vi "Teleop - Climb System (SubVI).vi"(0 "Driver Climb Activate":bool, 1 "Disabled":bool, 5 "Operator Climb Activate":bool, 7 "Desired cluster In":T3 {"shooterMotorMode" items=["PercentOutput"=0, "Position"=1, "Velocity"=2, "Current"=3, "Follower"=5, "MotionProfile"=6, "MotionMagic"=7, "MotionProfileArc"=10, "Disabled"=15]}, 9 "Constant Cluster in":T2 {"32. shooterHoodAngleRange" format="%_6f"; "31. turretAngleRange" format="%_6f"; "30. shooterVelocityLowerLimit" format="%_6f"; "29. shooterVelocityUpperLimit" format="%_6f"; "28. Robot Track Width (inches)" format="%_6f"; "27. Shooter Spin Up Speed (RPM)" format="%_6f"; "26. Climb Down Speed %" format="%_6f"; "25. Climb Up Speed %" format="%_6f"; "24. wallShooterVelocity" format="%_6f"; "23. Intake Spit Speed %" format="%_6f"; "22. Intake Suck Speed %" format="%_6f"; "21. CP Wheel Diameter" format="%_6f"; "20. Clockwise CP Fudge" format="%_6f"; "19. CouterClockwise CP Fudge" format="%_6f"; "18. Inches per Sector" format="%_6f"; "17. Ticks/Rotation Neo 550" format="%_6f"; "16. Control Panel Wheel Diameter" format="%_6f"; "15. Center-Center Sector Distance" format="%_6f"; "14. Inches / Tick Drivetrain" format="%_6f"; "13. Auton I Output Limit Drive Straight Gain" format="%_6f"; "12. Auton Deriv Drive Straight Gain" format="%_6f"; "11. Auton Int Drive Straight Gain" format="%_6f"; "10. Auton Prop Drive Straight Gain" format="%_6f"; "9. Auton I Output Limit Turn Gain" format="%_6f"; "8. Auton Deriv Turn Gain" format="%_6f"; "7. Auton Int Turn Gain" format="%_6f"; "1. Auton Prop Drive Gain" format="%_6f"; "2. Auton Int Drive Gain" format="%_6f"; "3. Auton Deriv Drive Gain" format="%_6f"; "4. I Output Drive  Limit" format="%_6f"; "5. Auto Drive Cheat (%)" format="%_6f"; "6. Auton Prop Turn Gain" format="%_6f"}, 11 "Climb Up":bool, 12 "Sensors In":T1) -> (8 "Desired cluster Out":T3 {"shooterMotorMode" items=["PercentOutput"=0, "Position"=1, "Velocity"=2, "Current"=3, "Follower"=5, "MotionProfile"=6, "MotionMagic"=7, "MotionProfileArc"=10, "Disabled"=15]}, 10 "Constant Cluster out":T2 {"32. shooterHoodAngleRange" format="%_6f"; "31. turretAngleRange" format="%_6f"; "30. shooterVelocityLowerLimit" format="%_6f"; "29. shooterVelocityUpperLimit" format="%_6f"; "28. Robot Track Width (inches)" format="%_6f"; "27. Shooter Spin Up Speed (RPM)" format="%_6f"; "26. Climb Down Speed %" format="%_6f"; "25. Climb Up Speed %" format="%_6f"; "24. wallShooterVelocity" format="%_6f"; "23. Intake Spit Speed %" format="%_6f"; "22. Intake Suck Speed %" format="%_6f"; "21. CP Wheel Diameter" format="%_6f"; "20. Clockwise CP Fudge" format="%_6f"; "19. CouterClockwise CP Fudge" format="%_6f"; "18. Inches per Sector" format="%_6f"; "17. Ticks/Rotation Neo 550" format="%_6f"; "16. Control Panel Wheel Diameter" format="%_6f"; "15. Center-Center Sector Distance" format="%_6f"; "14. Inches / Tick Drivetrain" format="%_6f"; "13. Auton I Output Limit Drive Straight Gain" format="%_6f"; "12. Auton Deriv Drive Straight Gain" format="%_6f"; "11. Auton Int Drive Straight Gain" format="%_6f"; "10. Auton Prop Drive Straight Gain" format="%_6f"; "9. Auton I Output Limit Turn Gain" format="%_6f"; "8. Auton Deriv Turn Gain" format="%_6f"; "7. Auton Int Turn Gain" format="%_6f"; "1. Auton Prop Drive Gain" format="%_6f"; "2. Auton Int Drive Gain" format="%_6f"; "3. Auton Deriv Drive Gain" format="%_6f"; "4. I Output Drive  Limit" format="%_6f"; "5. Auto Drive Cheat (%)" format="%_6f"; "6. Auton Prop Turn Gain" format="%_6f"}, 14 "Climb is latched":bool, 15 "Sensors Out":T1)   [LabVIEW 2019]
uses:
  Disabled/Constant VI_s/Disabled - Constant Cluster Typedef.ctl
  Autonomous/TypeDefs/Sensor TypeDef.ctl
  Desired Cluster.ctl
  <vilib>/Rock Robotics/WPI/ThirdParty/Phoenix-LabVIEW/Motor Controller/Controls/CTRE_Phoenix_MotorControl_ControlMode.ctl
panel:
  # "Inputs"
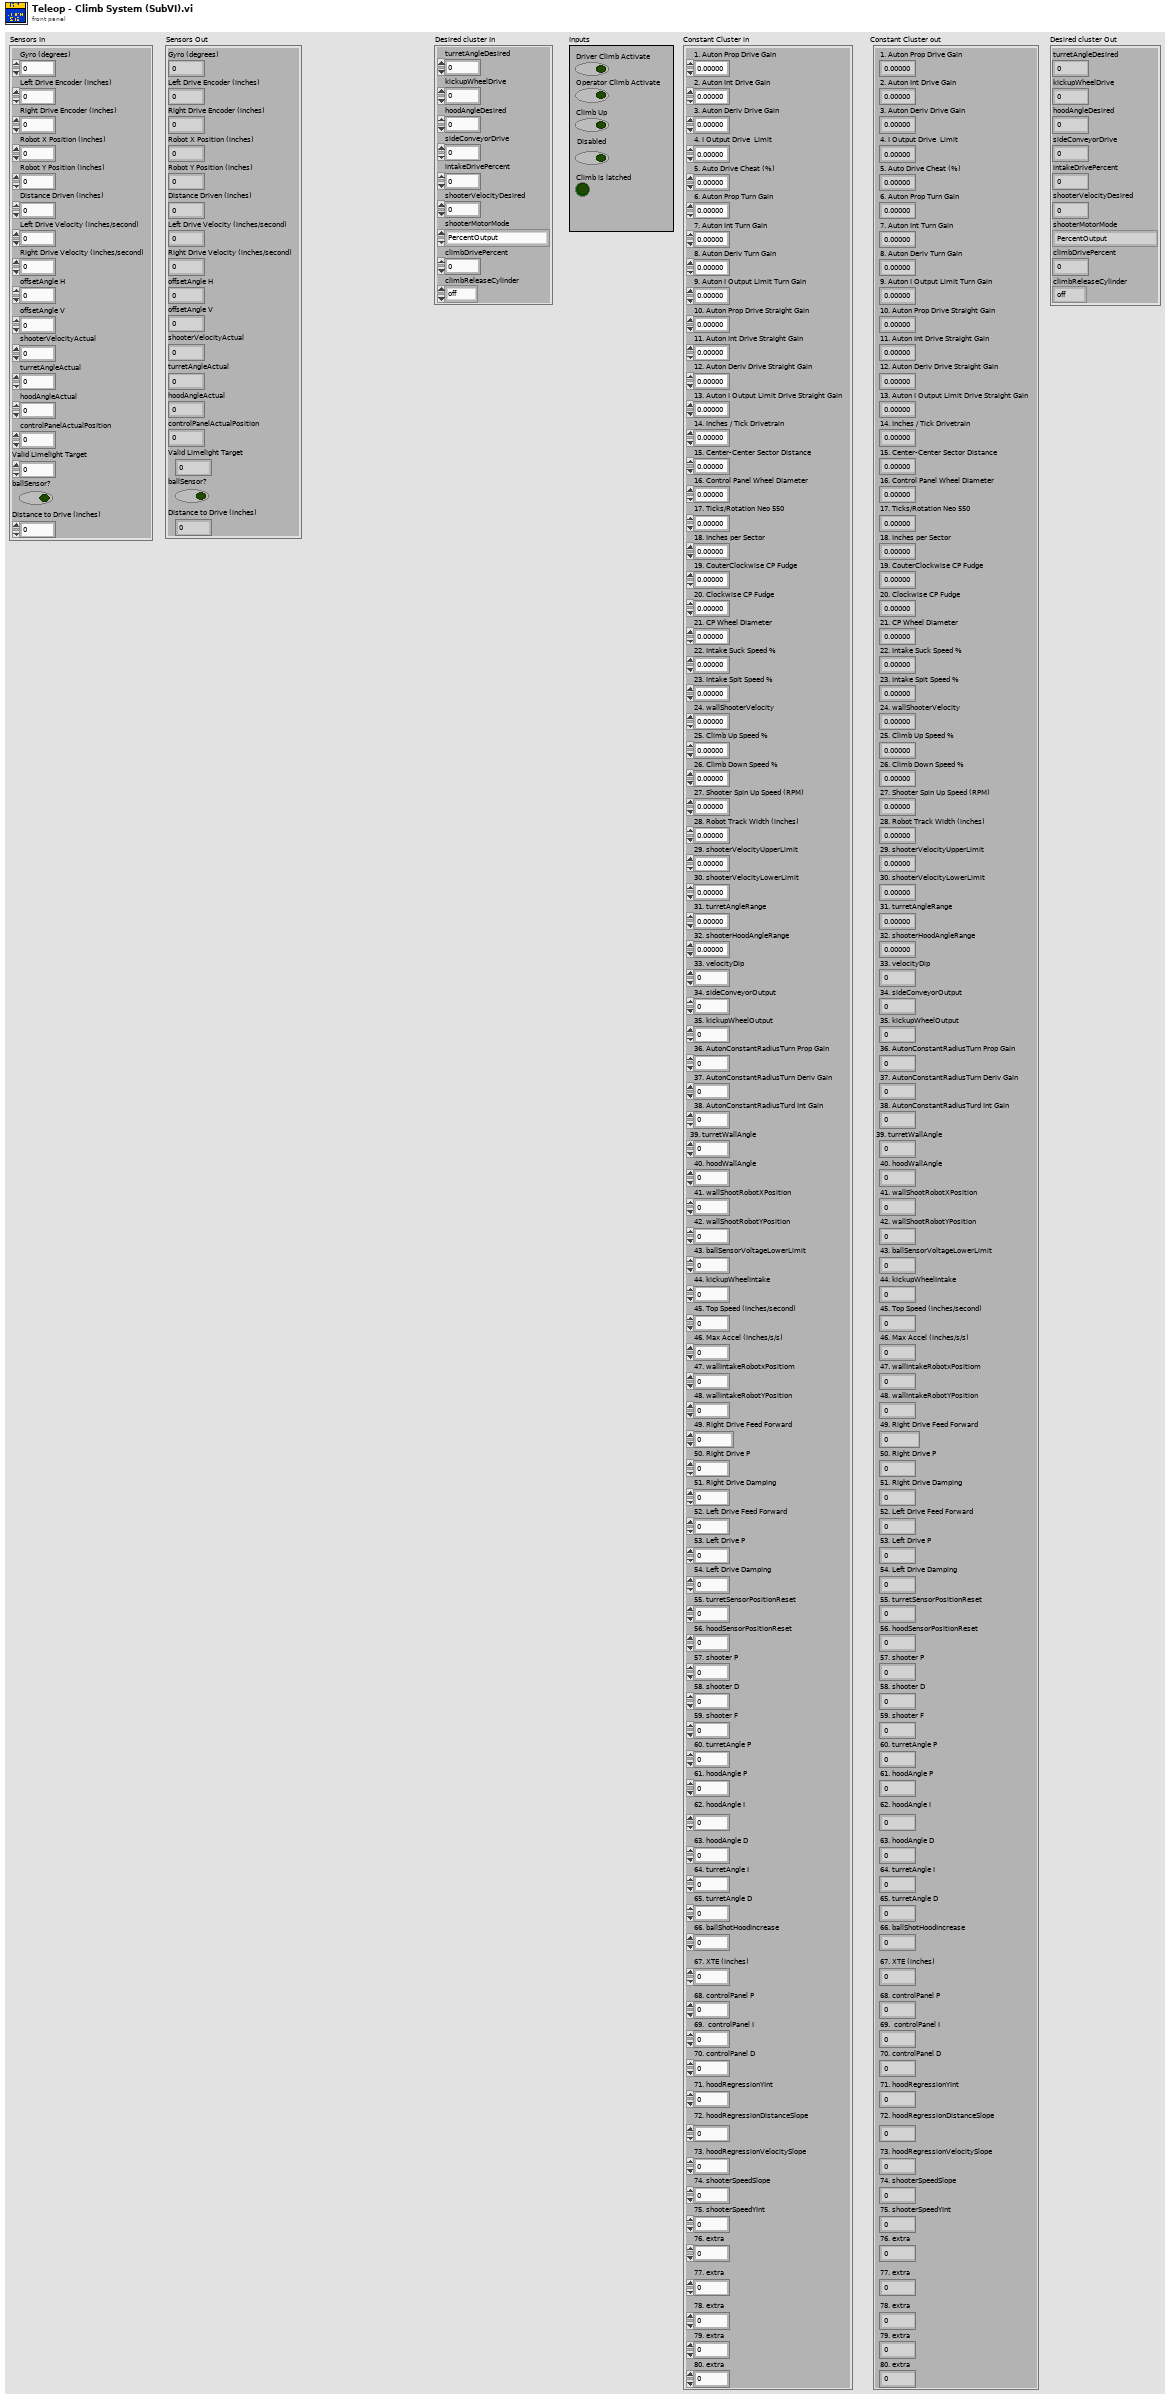
[diagram p1: front panel]
types:
  T1 = typedef "Sensor TypeDef.ctl" = cluster{"Gyro (degrees)":dbl, "Left Drive Encoder (inches)":dbl, "Right Drive Encoder (inches)":dbl, "Robot X Position (inches)":dbl, "Robot Y Position (inches)":dbl, "Distance Driven (inches)":dbl, "Left Drive Velocity (inches/second)":dbl, "Right Drive Velocity (inches/second)":dbl, "offsetAngle H":dbl, "offsetAngle V":dbl, "shooterVelocityActual":dbl, "turretAngleActual":dbl, "hoodAngleActual":dbl, "controlPanelActualPosition":dbl, "Valid Limelight Target":dbl, "ballSensor?":bool, "Distance to Drive (inches)":dbl}
  T2 = typedef "Disabled - Constant Cluster Typedef.ctl" = cluster{"1. Auton Prop Drive Gain":dbl, "2. Auton Int Drive Gain":dbl, "3. Auton Deriv Drive Gain":dbl, "4. I Output Drive  Limit":dbl, "5. Auto Drive Cheat (%)":dbl, "6. Auton Prop Turn Gain":dbl, "7. Auton Int Turn Gain":dbl, "8. Auton Deriv Turn Gain":dbl, "9. Auton I Output Limit Turn Gain":dbl, "10. Auton Prop Drive Straight Gain":dbl, "11. Auton Int Drive Straight Gain":dbl, "12. Auton Deriv Drive Straight Gain":dbl, "13. Auton I Output Limit Drive Straight Gain":dbl, "14. Inches / Tick Drivetrain":dbl, "15. Center-Center Sector Distance":dbl, "16. Control Panel Wheel Diameter":dbl, "17. Ticks/Rotation Neo 550":dbl, "18. Inches per Sector":dbl, "19. CouterClockwise CP Fudge":dbl, "20. Clockwise CP Fudge":dbl, "21. CP Wheel Diameter":dbl, "22. Intake Suck Speed %":dbl, "23. Intake Spit Speed %":dbl, "24. wallShooterVelocity":dbl, "25. Climb Up Speed %":dbl, "26. Climb Down Speed %":dbl, "27. Shooter Spin Up Speed (RPM)":dbl, "28. Robot Track Width (inches)":dbl, "29. shooterVelocityUpperLimit":dbl, "30. shooterVelocityLowerLimit":dbl, "31. turretAngleRange":dbl, "32. shooterHoodAngleRange":dbl, "33. velocityDip":dbl, "34. sideConveyorOutput":dbl, "35. kickupWheelOutput":dbl, "36. AutonConstantRadiusTurn Prop Gain":dbl, "37. AutonConstantRadiusTurn Deriv Gain":dbl, "38. AutonConstantRadiusTurd Int Gain":dbl, "39. turretWallAngle":dbl, "40. hoodWallAngle":dbl, "41. wallShootRobotXPosition":dbl, "42. wallShootRobotYPosition":dbl, "43. ballSensorVoltageLowerLimit":dbl, "44. kickupWheelIntake":dbl, "45. Top Speed (inches/second)":dbl, "46. Max Accel (inches/s/s)":dbl, "47. wallIntakeRobotxPositiom":dbl, "48. wallIntakeRobotYPosition":dbl, "49. Right Drive Feed Forward":dbl, "50. Right Drive P":dbl, "51. Right Drive Damping":dbl, "52. Left Drive Feed Forward":dbl, "53. Left Drive P":dbl, "54. Left Drive Damping":dbl, "55. turretSensorPositionReset":dbl, "56. hoodSensorPositionReset":dbl, "57. shooter P":dbl, "58. shooter D":dbl, "59. shooter F":dbl, "60. turretAngle P":dbl, "61. hoodAngle P":dbl, "62. hoodAngle I":dbl, "63. hoodAngle D":dbl, "64. turretAngle I":dbl, "65. turretAngle D":dbl, "66. ballShotHoodIncrease":dbl, "67. XTE (inches)":dbl, "68. controlPanel P":dbl, "69.  controlPanel I":dbl, "70. controlPanel D":dbl, "71. hoodRegressionYInt":dbl, "72. hoodRegressionDistanceSlope":dbl, "73. hoodRegressionVelocitySlope":dbl, "74. shooterSpeedSlope":dbl, "75. shooterSpeedYInt":dbl, "76. extra":dbl, "77. extra":dbl, "78. extra":dbl, "79. extra":dbl, "80. extra":dbl}
  T3 = typedef "Desired Cluster.ctl" = cluster{"turretAngleDesired":dbl, "kickupWheelDrive":dbl, "hoodAngleDesired":dbl, "sideConveyorDrive":dbl, "intakeDrivePercent":dbl, "shooterVelocityDesired":dbl, "shooterMotorMode":T4, "climbDrivePercent":dbl, "climbReleaseCylinder":enum16{"off", "on", "forward", "back"}}
  T4 = typedef "CTRE_Phoenix_MotorControl_ControlMode.ctl" = u16
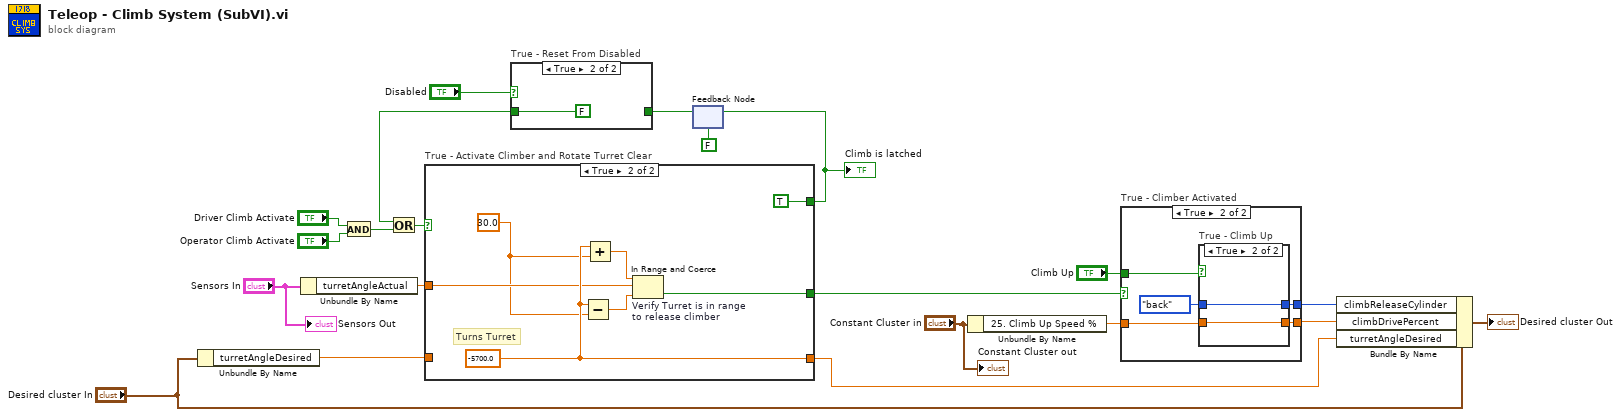
[diagram p0: block diagram]
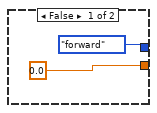
[diagram p3: hidden frame]
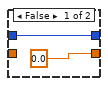
[diagram p4: hidden frame]
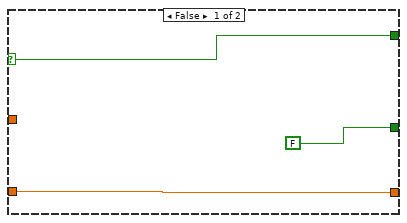
[diagram p5: hidden frame]
diagram:
  n1 = Unbundle By Name("Desired cluster In") -> ("turretAngleDesired"=w8:dbl)
  n2 = Unbundle By Name("Sensors In") -> ("turretAngleActual"=w10:dbl)
  n3 = And(x="Driver Climb Activate", y="Operator Climb Activate") -> (x .and. y?=w15:bool)
  n4 = feedback #1(FALSE) -> (w13:bool)
  n5 = case "True - Reset From Disabled" shown="True" "Disabled" {
    tunnel: w13 -> [w22 _]
    tunnel: [w22 FALSE] -> w12
    frame False {
    }
    frame True {
    }
  }
  n6 = Or(x=w12, y=w15) -> (x .or. y?=w17:bool)
  n7 = case "True - Activate Climber and Rotate Turret Clear" shown="True" w17 {
    selector: w17 -> [w26 _]
    tunnel: [w26 TRUE] -> w16
    tunnel: w8 -> [w25 _]
    tunnel: [w25 w30] -> w3
    tunnel: w10 -> [_ w29]
    tunnel: [FALSE w28] -> w9
    frame False {
    }
    frame True {
      w27 = 30.0 ("y")
      w30 = -5700.0 ("Turret In")
      # "Turns Turret"
      n8 = Subtract(x=w30, y=w27) -> (x-y=w31:dbl)
      n9 = Add(x=w30, y=w27) -> (x+y=w32:dbl)
      n10 = In Range and Coerce "Verify Turret is in range\nto release climber"(upper limit=w32, x=w29, lower limit=w31) -> (In Range?=w28:bool)  [unwired: 1 out]
    }
  }
  "Climb is latched" <- w16
  n11 = feedback-in #1(w16) -> ()
  n12 = Unbundle By Name("Constant Cluster in") -> ("25. Climb Up Speed %"=w18:dbl)
  n13 = case "True - Climber Activated" shown="True" w9 {
    tunnel: [0.0 ("controlPanel/climb") w39] -> w4
    tunnel: "Climb Up" -> [_ w40]
    tunnel: w18 -> [_ w38]
    tunnel: [enum16{"off", "on", "forward", "back"}."forward" ("climbReleaseCylinder") w37] -> w5
    frame False {
    }
    frame True {
      n14 = case "True - Climb Up" shown="True" w40 {
        tunnel: [0.0 ("26. Climb Down") w44] -> w39
        tunnel: w38 -> [_ w44]
        tunnel: [w41 w43] -> w37
        tunnel: enum16{"off", "on", "forward", "back"}."back" ("climbReleaseCylinder") -> [w41 w43]
        frame False {
        }
        frame True {
        }
      }
    }
  }
  n15 = Bundle By Name(cluster="Desired cluster In", "climbReleaseCylinder"=w5, "climbDrivePercent"=w4, "turretAngleDesired"=w3) -> (→"Desired cluster Out":T3)
  "Constant Cluster out" <- "Constant Cluster in"
  "Sensors Out" <- "Sensors In"
